vi "prompt_generation.vi"(8 "error in (no error)":errorcluster) -> (0 "error out":errorcluster, 3 "prompt":string)   [LabVIEW 2020]
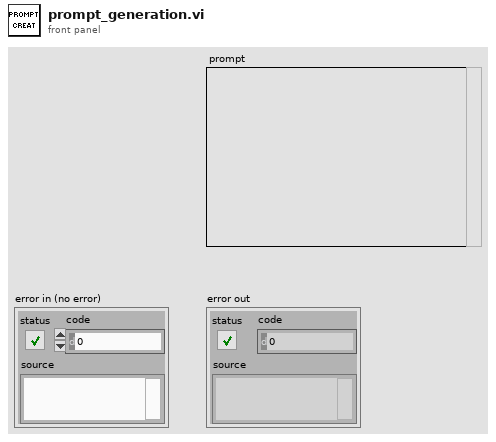
[diagram p1: front panel]
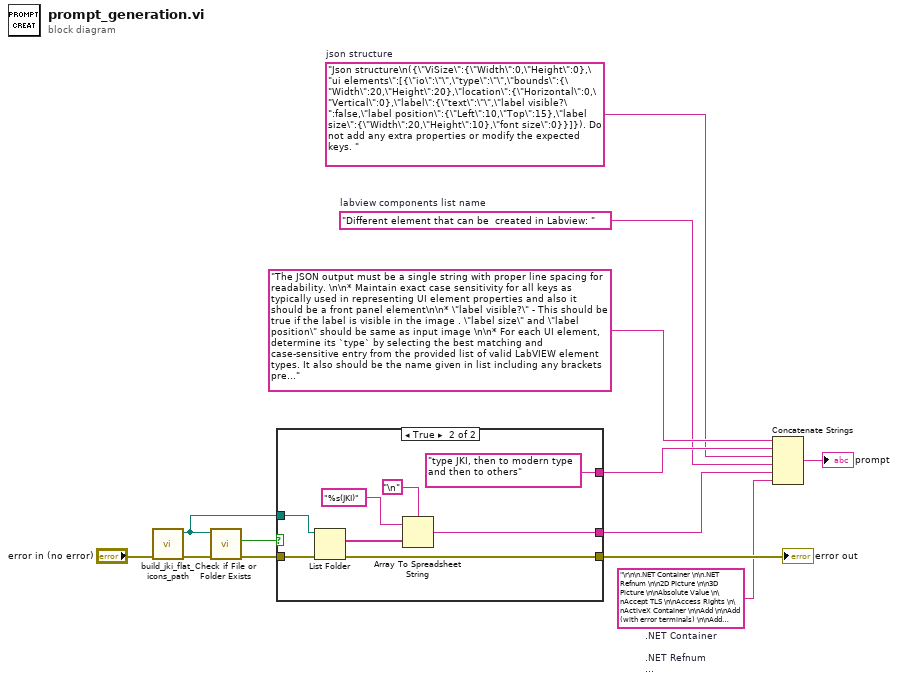
[diagram p0: block diagram]
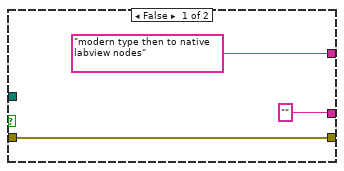
[diagram p2: hidden frame]
diagram:
  w4 = "\r\n\n.NET Container \n\n.NET Refnum \n\n2D Picture \n\n3D Picture \n\nAbsolute Value \n\nAccept TLS \n\nAccess Rights \n\nActiveX Container \n\nAdd \n\nAdd (with error terminals) \n\nAdd Array Elements \n\nAdd Entropy \n\nAdd Private Key To TLS Configuration \n\nAdd Trusted Certificate To TLS Configuration \n\nAgitator \n\nAllSpoll \n\nAlways Copy \n\nAnd \n\nAnd Array Elements \n\nAppend True/False String \n\nApplication Refnum \n\nArray (block diagram constant) \n\nArray (classic) \n\nArray (modern) \n\nArray Interface Control \n\nArray Max & Min \n\nArray of Strings to Path \n\nArray Size \n\nArray Subset \n\nArray To Cluster \n\nArray To Spreadsheet String \n\nArrayMemInfo \n\nAssert Structural Type Match \n\nAssert Structural Type Mismatch \n\nAtmospheric Tank (classic) \n\nAtmospheric Tank (modern) \n\nAutomation Close \n\nAutomation Open \n\nAutomation Refnum \n\nAvogadro Constant (1/mol) \n\nBase 10 Logarithm Of e \n\nBin #1 \n\nBin #2 \n\nBitpack to Array \n\nBluetooth Close Connection \n\nBluetooth Create Listener \n\nBluetooth Discover \n\nBluetooth Network Connection Refnum \n\nBluetooth Open Connection \n\nBluetooth Read \n\nBluetooth Wait On Listener \n\nBluetooth Write \n\nBoolean Array To Number \n\nBoolean To (0,1) \n\nBuild Array \n\nBuild Cluster Array \n\nBuild Map \n\nBuild Matrix \n\nBuild Path \n\nBuild Set \n\nBuild Waveform \n\nBundle \n\nBundle By Name \n\nByte Array To String \n\nByte Array To UTF-8 String \n\nByte Stream File Refnum \n\nCall By Reference \n\nCall Chain \n\nCall Library Function Node \n\nCall Parent Class Method \n\nCAN Channel (block diagram constant) \n\nCAN Channel (classic) \n\nCAN Channel (modern) \n\nCAN Channel (system) \n\nCAN Interface (block diagram constant) \n\nCAN Interface (classic) \n\nCAN Interface (modern) \n\nCAN Interface (system) \n\nCAN Task (block diagram constant) \n\nCAN Task (classic) \n\nCAN Task (modern) \n\nCAN Task (system) \n\nCancel Button (modern) \n\nCancel Button (system) \n\nCancel Notification \n\nCarriage Return Constant \n\nCase Structure \n\nCast Unit Bases \n\nCheck Valve \n\nCheckbox (classic) \n\nCheckBox (modern) \n\nCheckbox (system) \n\nClass Specifier Constant \n\nClassic Color Box \n\nClassic Color Ramp \n\nClassic Horizontal Slide Switch \n\nClassic Vertical Slide \n\nClear Fixed-Point Overflow Status \n\nClose File \n\nClose File (deprecated) \n\nClose Python Session \n\nClose Reference \n\nClose TLS Configuration \n\nClose Variable Connection \n\nClosure Structure \n\nCluster (classic) \n\nCluster (modern) \n\nCluster Constant \n\nCluster To Array \n\nCode Interface Node \n\nCoerce To Type \n\nCollection Size \n\nColor Box Constant \n\nColor Box Thin Border \n\nColored Rectangle (broken?) \n\nCombo Box (classic) \n\nCombo Box (modern) \n\nCombo Box (system) \n\nCombo Box Constant \n\nComplex Conjugate \n\nComplex To Polar \n\nComplex To Re/Im \n\nCompound Arithmetic \n\nCompressor \n\nConcatenate Strings \n\nConditional Disable Structure \n\nConstructor Node \n\nControl & Simulation Loop \n\nControl Help Window \n\nControl Online Help \n\nControl Refnum \n\nConvert Unit \n\nConveyer \n\nCopy \n\nCopy (deprecated) \n\nCosecant \n\nCosine \n\nCotangent \n\nCPU Information \n\nCreate Folder \n\nCreate Network Stream Endpoint \n\nCreate Network Stream Reader Endpoint \n\nCreate Network Stream Writer Endpoint \n\nCreate Stream \n\nCreate Unique Network Stream Endpoint \n\nCreate Unique Network Stream Reader Endpoint \n\nCreate Unique Network Stream Writer Endpoint \n\nCreate User Event \n\nCurrent Processor ID \n\nCurrent VI's Menubar \n\nCurrent VI's Path \n\nDAQmx Analog Trigger Source (block diagram constant) \n\nDAQmx Analog Trigger Source (classic) \n\nDAQmx Analog Trigger Source (modern) \n\nDAQmx Analog Trigger Source (system) \n\nDAQmx Device Name (block diagram constant) \n\nDAQmx Device Name (classic) \n\nDAQmx Device Name (modern) \n\nDAQmx Device Name (system) \n\nDAQmx Global Channel (block diagram constant) \n\nDAQmx Global Channel (classic) \n\nDAQmx Global Channel (modern) \n\nDAQmx Global Channel (system) \n\nDAQmx Physical Channel (block diagram constant) \n\nDAQmx Physical Channel (classic) \n\nDAQmx Physical Channel (modern) \n\nDAQmx Physical Channel (system) \n\nDAQmx Scale Name (block diagram constant) \n\nDAQmx Scale Name (classic) \n\nDAQmx Scale Name (modern) \n\nDAQmx Scale Name (system) \n\nDAQmx Switch (block diagram constant) \n\nDAQmx Switch (classic) \n\nDAQmx Switch (modern) \n\nDAQmx Switch (system) \n\nDAQmx Task Name (block diagram constant) \n\nDAQmx Task Name (classic) \n\nDAQmx Task Name (modern) \n\nDAQmx Task Name (system) \n\nDAQmx Terminal (block diagram constant) \n\nDAQmx Terminal (classic) \n\nDAQmx Terminal (modern) \n\nDAQmx Terminal (system) \n\nData Cache Size \n\nData Log File Refnum \n\nData Value Reference \n\nData Value Reference Constant \n\nDataSocket Close \n\nDataSocket Open \n\nDataSocket Read \n\nDataSocket Refnum \n\nDataSocket Write \n\nDate/Time To Seconds \n\nDecimal Digit? \n\nDecimal String To Number \n\nDecimate 1D Array \n\nDecomposeLockDataValRef \n\nDecomposeVariant \n\nDecrement \n\nDefault Directory \n\nDelete \n\nDelete (deprecated) \n\nDelete Data Value Reference \n\nDelete From Array \n\nDelete Menu Items \n\nDelete Variant Attribute \n\nDelete Waveform Attribute \n\nDeny Access \n\nDequeue Element \n\nDestroy Stream Endpoint \n\nDestroy User Event \n\nDevClear \n\nDevClearList \n\nDevice Control/Status \n\nDevice Refnum \n\nDiagram Disable Structure \n\nDial (classic) \n\nDial (modern) \n\nDigital Data (classic) \n\nDigital Data (modern) \n\nDigital Waveform Graph (classic) \n\nDigital Waveform Graph (modern) \n\nDirect Variable Read \n\nDirect Variable Write \n\nDivide \n\nDivide (with error terminals) \n\nDlg Horiz Scrollbar \n\nDlg Mac Group Box \n\nDlg Numeric #1 \n\nDlg Numeric #2 \n\nDlg String \n\nDlg Vert Scrollbar \n\nDown Arrow \n\nDown Bow Valve (flat) \n\nDown Bow Valve (outline) \n\nDown Bow Valve (shaded) \n\nDown Rect Valve (flat) \n\nDown Rect Valve (outline) \n\nDown Rect Valve (shaded) \n\nDown Tee (flat) \n\nDown Tee (shaded) \n\nDynamic FPGA Interface Cast \n\nEased Corner Rectangle \n\nElement of Set? \n\nElementary Charge (C) \n\nEmpty Array? \n\nEmpty Collection? \n\nEmpty Path Constant \n\nEmpty String Constant \n\nEmpty String/Path? \n\nEnable Menu Tracking \n\nEnableLocal \n\nEnableRemote \n\nEnd of Line Constant \n\nEnqueue Element \n\nEnqueue Element At Opposite End \n\nEnum (classic) \n\nEnum (modern) \n\nEnum (system) \n\nEnum Constant \n\nEOF \n\nEqual To 0? \n\nEqual? \n\nError Ring Constant \n\nEvent Callback Refnum \n\nEvent Data Node \n\nEvent Structure \n\nExchanger \n\nExclusive Or \n\nExponential \n\nExponential (Arg) -1 \n\nExpression Node \n\nFalse Constant \n\nFeedback Node \n\nFieldPoint IO Point (block diagram constant) \n\nFieldPoint IO Point (classic) \n\nFieldPoint IO Point (modern) \n\nFIFO Refnum \n\nFile Dialog \n\nFile Dialog (deprecated) \n\nFile Path Control (classic) \n\nFile Path Control (modern) \n\nFile Path Control (system) \n\nFile Path Indicator (classic) \n\nFile Path Indicator (modern) \n\nFile/Directory Info \n\nFile/Directory Info (deprecated) \n\nFindLstn \n\nFindRQS \n\nFirst Call? \n\nFixed-Point Overflow? \n\nFixed-Point to Integer Cast \n\nFlat Box \n\nFlat Circle \n\nFlat Down Triangle \n\nFlat Frame \n\nFlat Left Triangle \n\nFlat Right Triangle \n\nFlat Round Button \n\nFlat Rounded Box \n\nFlat Sequence Structure \n\nFlat Square Button \n\nFlat Up Triangle \n\nFlatten To JSON \n\nFlatten To String \n\nFlatten To XML \n\nFlattened String To Variant \n\nFloating Point Equal? \n\nFlush Event Queue \n\nFlush File \n\nFlush File (deprecated) \n\nFlush Queue \n\nFlush Stream \n\nFor Loop \n\nFork \n\nFormat Date/Time String \n\nFormat Into File \n\nFormat Into String \n\nFormat Value \n\nFormula Node \n\nFPGA Refnum to Session \n\nFract/Exp String To Number \n\nFramed Color Box (classic) \n\nFramed Color Box (modern) \n\nFree Label \n\nFurnace \n\nGauge (classic) \n\nGauge (modern) \n\nGauge for Simon \n\nGenerate Front Panel Activity \n\nGenerate Occurrence \n\nGenerate User Event \n\nGenerate User-Defined Trace Event \n\nGet Control Values by Index \n\nGet Datalog Position \n\nGet Date/Time In Seconds \n\nGet Date/Time String \n\nGet Drag Drop Data \n\nGet File Position \n\nGet File Size \n\nGet Fixed-Point Components \n\nGet Help Window Status \n\nGet Matrix Diagonal \n\nGet Matrix Elements \n\nGet Menu Item Info \n\nGet Menu Selection \n\nGet Menu Short Cut Info \n\nGet Notifier Status \n\nGet Number of Records \n\nGet Permissions \n\nGet Queue Status \n\nGet Submatrix \n\nGet Type and Creator \n\nGet Variant Attribute \n\nGet Volume Info \n\nGet Waveform Attribute \n\nGet Waveform Components \n\nGlobal Variable \n\nGPIB Clear \n\nGPIB Initialization \n\nGPIB Misc \n\nGPIB Read \n\nGPIB Serial Poll \n\nGPIB Status \n\nGPIB Trigger \n\nGPIB Wait \n\nGPIB Write \n\nGravitational Constant (N m2/kg2) \n\nGreater Or Equal To 0? \n\nGreater Or Equal? \n\nGreater Than 0? \n\nGreater? \n\nHandle Peek \n\nHandle Poke \n\nHex Digit? \n\nHexadecimal String To Number \n\nHopper #1 \n\nHopper #2 \n\nHoriz Line \n\nHoriz Pipe (flat) \n\nHoriz Pipe (shaded) \n\nHorizontal Button Box \n\nHorizontal Fill Slide (classic) \n\nHorizontal Fill Slide (modern) \n\nHorizontal Gradient Oval \n\nHorizontal Gradient Rectangle \n\nHorizontal Gradient Rounded Rectangle \n\nHorizontal Graduated Bar \n\nHorizontal Pointer Slide (classic) \n\nHorizontal Pointer Slide (modern) \n\nHorizontal Pointer Slide (system) \n\nHorizontal Progress Bar (modern) \n\nHorizontal Progress Bar (system) \n\nHorizontal Scrollbar \n\nHorizontal Slide (classic) \n\nHorizontal Slide (system) \n\nHorizontal Smooth Box \n\nHorizontal Splitter Bar \n\nHorizontal Splitter Bar (Classic) \n\nHorizontal Splitter Bar (NXG Style) \n\nHorizontal Splitter Bar (System) \n\nHorizontal Switch \n\nHorizontal Tank \n\nHorizontal Toggle Switch (classic) \n\nHorizontal Toggle Switch (modern) \n\nHyperbolic Cosecant \n\nHyperbolic Cosine \n\nHyperbolic Cotangent \n\nHyperbolic Secant \n\nHyperbolic Sine \n\nHyperbolic Tangent \n\nIMAQ Session \n\nImplies \n\nIn Place Element Structure \n\nIn Range and Coerce \n\nInclude Fixed-Point Overflow Status \n\nIncrement \n\nIndex & Bundle Cluster Array \n\nIndex Array \n\nIndex String Array \n\nInitialize Array \n\nInline C Node \n\nInsert Into Array \n\nInsert Into Map \n\nInsert Into Set \n\nInsert Menu Items \n\nInteger to Fixed-Point Cast \n\nIntensity Chart (classic) \n\nIntensity Chart (modern) \n\nIntensity Graph (classic) \n\nIntensity Graph (modern) \n\nInterleave 1D Arrays \n\nInterpolate 1D Array \n\nInverse Cosecant \n\nInverse Cosine \n\nInverse Cotangent \n\nInverse Hyperbolic Cosecant \n\nInverse Hyperbolic Cosine \n\nInverse Hyperbolic Cotangent \n\nInverse Hyperbolic Secant \n\nInverse Hyperbolic Sine \n\nInverse Hyperbolic Tangent \n\nInverse Secant \n\nInverse Sine \n\nInverse Tangent \n\nInverse Tangent (2 Input) \n\nInvoke Node \n\nIP To String \n\nIrDA Close Connection \n\nIrDA Create Listener \n\nIrDA Discover \n\nIrDA Network Connection Refnum \n\nIrDA Open Connection \n\nIrDA Read \n\nIrDA Wait On Listener \n\nIrDA Write \n\nIsDebuggingActive \n\nIVI Delete Session \n\nIVI Logical Name (block diagram constant) \n\nIVI Logical Name (classic) \n\nIVI Logical Name (modern) \n\nIVI New Session \n\nJoin \n\nJoin Numbers \n\nJunction \n\nKnob (classic) \n\nKnob (modern) \n\nLabel (modern) \n\nLabel (system) \n\nLabeled Oblong Button \n\nLabeled Rectangular Button \n\nLabeled Round Button \n\nLabeled Square Button \n\nLabVIEW Object \n\nLeak Variant Value Reference \n\nLED Button \n\nLeft Arrow \n\nLeft Bow Valve (flat) \n\nLeft Bow Valve (outline) \n\nLeft Bow Valve (shaded) \n\nLeft Down Elbow (flat) \n\nLeft Down Elbow (shaded) \n\nLeft Pump (flat) \n\nLeft Pump (shaded) \n\nLeft Rect Valve (flat) \n\nLeft Rect Valve (outline) \n\nLeft Rect Valve (shaded) \n\nLeft Tee (flat) \n\nLeft Tee (shaded) \n\nLeft Up Elbow (flat) \n\nLeft Up Elbow (shaded) \n\nLess Or Equal To 0? \n\nLess Or Equal? \n\nLess Than 0? \n\nLess? \n\nLexical Class \n\nLine (chiseled, system) \n\nLine (chiseled, thick) \n\nLine (chiseled, thin) \n\nLine (thick) \n\nLine (thin) \n\nLine Feed Constant \n\nLine with Arrow (thick) \n\nLine with Arrow (thin) \n\nList Directory \n\nList Folder \n\nListbox (classic) \n\nListbox (modern) \n\nListbox (system) \n\nListbox Symbol Ring Constant \n\nLoad Certificates Into Memory \n\nLoad Private Key Into Memory \n\nLocal Variable \n\nLock Range \n\nLogarithm Base 10 \n\nLogarithm Base 2 \n\nLogarithm Base X \n\nLogical Shift \n\nLook In Map \n\nLookup Channel Probe \n\nLossy Enqueue Element \n\nLowered Box (thick) \n\nLowered Rounded Box \n\nMachine Epsilon \n\nMake TLS Configuration Immutable \n\nMakeAddr \n\nMantissa & Exponent \n\nMap \n\nMap Constant \n\nMatch First String \n\nMatch Pattern \n\nMatch True/False String \n\nMathScript Call By Reference \n\nMathScript Node \n\nMATLAB script \n\nMatrix Size \n\nMax & Min \n\nMenu Refnum \n\nMenu Ring (classic) \n\nMenu Ring (modern) \n\nMenu-Popup Ring \n\nMerge Errors \n\nMerge Signals \n\nMeter (classic) \n\nMeter (modern) \n\nMixed Checkbox (system) \n\nMixed Signal Graph \n\nMolar Gas Constant (J/(mol K)) \n\nMotion Resource (block diagram constant) \n\nMotion Resource (classic) \n\nMotion Resource (modern) \n\nMotor (flat) \n\nMotor (shaded) \n\nMove \n\nMove (deprecated) \n\nMulti-Segment Pipe \n\nMulticolumn Listbox (classic) \n\nMulticolumn Listbox (modern) \n\nMulticolumn Listbox (system) \n\nMultiply \n\nMultiply (with error terminals) \n\nMultiply Array Elements \n\nMultirate Structure \n\nNatural Logarithm \n\nNatural Logarithm (Arg +1) \n\nNatural Logarithm Base \n\nNatural Logarithm Of 10 \n\nNatural Logarithm Of 2 \n\nNatural Logarithm Of Pi \n\nNegate \n\nNegative Infinity \n\nNew Data Value Reference \n\nNew Directory \n\nNew File \n\nNew TLS Configuration \n\nNew VI \n\nNew VI Object \n\nNot \n\nNot A Number/Path/Refnum? \n\nNot A Path Constant \n\nNot a Refnum Constant \n\nNot a Shared Variable \n\nNot And \n\nNot Equal To 0? \n\nNot Equal? \n\nNot Exclusive Or \n\nNot Or \n\nNotifier Refnum \n\nNumber of Cache Levels \n\nNumber To Boolean Array \n\nNumber To Decimal String \n\nNumber To Engineering String \n\nNumber To Exponential String \n\nNumber To Fractional String \n\nNumber To Hexadecimal String \n\nNumber To Octal String \n\nNumeric Constant \n\nNumeric Control (classic) \n\nNumeric Control (modern) \n\nNumeric Control (system) \n\nNumeric Indicator (classic) \n\nNumeric Indicator (modern) \n\nObtain Notifier \n\nObtain Queue \n\nOccurrence Refnum \n\nOctal Digit? \n\nOctal String To Number \n\nOK Button (modern) \n\nOK Button (system) \n\nOld VISA Open \n\nOLE Variant \n\nOne Button Dialog \n\nOpen and Verify Variable Connection \n\nOpen Application Reference \n\nOpen Device \n\nOpen Dynamic Bitfile Reference \n\nOpen File \n\nOpen Python Session \n\nOpen Tank (flat classic) \n\nOpen Tank (shaded classic) \n\nOpen Variable Connection \n\nOpen Variable Connection in Background \n\nOpen VI Object Reference \n\nOpen VI Reference \n\nOpen/Create/Replace Datalog \n\nOpen/Create/Replace File \n\nOr \n\nOr Array Elements \n\nOval with Shadow \n\nPackage Matrix \n\nPassControl \n\nPath Constant \n\nPath to Array of Strings \n\nPath To String \n\nPath Type \n\nPi \n\nPi Divided By 2 \n\nPi Multiplied By 2 \n\nPick Line \n\nPict Ring (classic) \n\nPict Ring (modern) \n\nPict Ring (system) \n\nPixMap \n\nPixMap (warning: dangerous) \n\nPlanck's Constant (J/Hz) \n\nPlatform Flat Square Button \n\nPlug-In Control \n\nPolar To Complex \n\nPolar To Re/Im \n\nPositive Infinity \n\nPower Of 10 \n\nPower Of 2 \n\nPower Of X \n\nPPoll \n\nPPollConfig \n\nPPollUnconfig \n\nPreallocated Read from Binary File \n\nPreserve Run-Time Class \n\nPressure Tank (flat) \n\nPressure Tank (shaded) \n\nPreview Queue Element \n\nPrintable? \n\nProperty Node \n\nPulldown Menu Ring \n\nPush Button \n\nPython Node \n\nPython Session Refnum \n\nQueue Refnum \n\nQuit LabVIEW \n\nQuotient & Remainder \n\nRace Structure \n\nRadio Button (system) \n\nRadio Buttons (classic) \n\nRadio Buttons (modern) \n\nRadio Buttons (system) \n\nRaised Box (classic) \n\nRaised Box (modern) \n\nRaised Circle \n\nRaised Down Triangle \n\nRaised Frame \n\nRaised Left Triangle \n\nRaised Right Triangle \n\nRaised Rounded Box \n\nRaised Up Triangle \n\nRandom Number (0-1) \n\nRcvRespMsg \n\nRe-accept TLS \n\nRe/Im To Complex \n\nRe/Im To Polar \n\nRead Datalog \n\nRead Device \n\nRead File \n\nRead from Binary File \n\nRead from Text File \n\nRead Map Max & Min Keys \n\nRead Multiple Elements from Stream \n\nRead Set Max & Min \n\nRead Single Element from Stream \n\nRead Variable \n\nRead Variable with Timeout \n\nReadStatus \n\nReceive \n\nReceiveSetup \n\nRecessed Box \n\nRecessed Circle \n\nRecessed Down Triangle \n\nRecessed Frame (modern) \n\nRecessed Frame (system) \n\nRecessed Left Triangle \n\nRecessed Menu Ring \n\nRecessed Right Triangle \n\nRecessed Rounded Box \n\nRecessed Up Triangle \n\nReciprocal \n\nReciprocal Of e \n\nReciprocal Of Pi \n\nRecomposeUnlockDataValRef (warning: dangerous) \n\nRecomposeVariant (warning: dangerous) \n\nRectangular Stop Button \n\nRefnum to Path \n\nRefnum to Session \n\nRegion \n\nRegister Event Callback \n\nRegister For Events \n\nRegister Session \n\nRelease Notifier \n\nRelease Queue \n\nRemove Fixed-Point Overflow Status \n\nRemove From Map \n\nRemove From Set \n\nReplace Array Subset \n\nReplace Substring \n\nRequest Deallocation \n\nResetSys \n\nReshape Array \n\nResize Matrix \n\nResource Index \n\nReverse 1D Array \n\nReverse String \n\nRight Arrow \n\nRight Bow Valve (flat) \n\nRight Bow Valve (outline) \n\nRight Bow Valve (shaded) \n\nRight Down Elbow (flat) \n\nRight Down Elbow (shaded) \n\nRight Pump (flat) \n\nRight Pump (shaded) \n\nRight Rect Valve (flat) \n\nRight Rect Valve (outline) \n\nRight Rect Valve (shaded) \n\nRight Tee (flat) \n\nRight Tee (shaded) \n\nRight Up Elbow (flat) \n\nRight Up Elbow (shaded) \n\nRocker \n\nRotary Feeder \n\nRotate \n\nRotate 1D Array \n\nRotate Left With Carry \n\nRotate Right With Carry \n\nRotate String \n\nRound Button \n\nRound LED (classic) \n\nRound LED (modern) \n\nRound Light \n\nRound Push Button \n\nRound Push Button (profile) \n\nRound Radio Button \n\nRound Stop Button \n\nRound To Nearest \n\nRound Toward +Infinity \n\nRound Toward -Infinity \n\nRounded Rectangle with Shadow \n\nRT FIFO Create \n\nRT FIFO Delete \n\nRT FIFO Read \n\nRT FIFO Write \n\nRydberg Constant (1/m) \n\nScale By Power Of 2 \n\nScan From File \n\nScan From String \n\nScan String For Tokens \n\nScan Value \n\nScanned Variable Read \n\nScanned Variable Write \n\nSearch 1D Array \n\nSearch and Replace String \n\nSearch Variable Container \n\nSearch/Split String \n\nSecant \n\nSeconds To Date/Time \n\nSeek \n\nSelect \n\nSend \n\nSend Notification \n\nSendCmds \n\nSendDataBytes \n\nSendIFC \n\nSendList \n\nSendLLO \n\nSendSetup \n\nSession to Refnum \n\nSet \n\nSet Constant \n\nSet Control Values by Index \n\nSet Datalog Position \n\nSet File Position \n\nSet File Size \n\nSet Matrix Diagonal \n\nSet Matrix Elements \n\nSet Menu Item Info \n\nSet Number of Records \n\nSet Occurrence \n\nSet Permissions \n\nSet Submatrix \n\nSet Type and Creator \n\nSet Variant Attribute \n\nSet Waveform Attribute \n\nSetRWLS \n\nSetTimeOut \n\nShared Variable \n\nShared Variable Constant \n\nShared Variable Control (classic) \n\nShared Variable Control (modern) \n\nShared Variable to String \n\nSign \n\nSimple Horizontal Slide \n\nSimple Numeric \n\nSimple String \n\nSimple Vertical Slide \n\nSinc \n\nSine \n\nSine & Cosine \n\nSize Handle \n\nSlide Switch \n\nSmoothed Oval \n\nSmoothed Rounded Rectangle \n\nSort 1D Array \n\nSort Array of String \n\nSpeed Of Light In Vacuum (m/sec) \n\nSpin Control (system) \n\nSplit 1D Array \n\nSplit Button \n\nSplit Number \n\nSplit Signals \n\nSpreadsheet String To Array \n\nSquare \n\nSquare Button \n\nSquare LED (classic) \n\nSquare LED (modern) \n\nSquare Light \n\nSquare Push Button \n\nSquare Push Button (profile) \n\nSquare Radio Button \n\nSquare Root \n\nStacked Sequence Structure \n\nStart TLS \n\nState \n\nState Diagram \n\nStatic VI Reference \n\nStop \n\nStop Button \n\nString Constant \n\nString Control (classic) \n\nString Control (modern) \n\nString Control (system) \n\nString Indicator (classic) \n\nString Indicator (modern) \n\nString Length \n\nString Subset \n\nString To Byte Array \n\nString To IP \n\nString To Path \n\nString to Shared Variable \n\nStrip Path \n\nSubPanel \n\nSubPanel (Classic) \n\nSubPanel (NXG Style) \n\nSubPanel (System) \n\nSubtract \n\nSubtract (with error terminals) \n\nSwap Bytes \n\nSwap Values \n\nSwap Vector Element \n\nSwap Words \n\nTab Constant \n\nTab Control (classic) \n\nTab Control (modern) \n\nTab Control (NXG Style) \n\nTab Control (system) \n\nTable (classic) \n\nTable (modern) \n\nTable (system) \n\nTag Attribute Ring \n\nTangent \n\nTank (classic) \n\nTank (modern) \n\nTarget Structure \n\nTCP Close Connection \n\nTCP Create Listener \n\nTCP Flattened Read \n\nTCP Flattened Write \n\nTCP Flex Read \n\nTCP Flex Write \n\nTCP Network Connection Refnum \n\nTCP Open Connection \n\nTCP Read \n\nTCP Wait On Listener \n\nTCP Write \n\nTDMS Advanced Asynchronous Read (Data Ref) \n\nTDMS Advanced Asynchronous Write (Data Ref) \n\nTDMS Close \n\nTDMS Configure Asynchronous Reads (Data Ref) \n\nTDMS Configure Asynchronous Writes (Data Ref) \n\nTDMS Defragment \n\nTDMS Delete Data \n\nTDMS File \n\nTDMS Flush \n\nTDMS Get Asynchronous Read Status (Data Ref) \n\nTDMS Get Asynchronous Write Status (Data Ref) \n\nTDMS Get Properties \n\nTDMS In Memory Close \n\nTDMS In Memory Open \n\nTDMS In Memory Read Bytes \n\nTDMS List Contents \n\nTDMS Open \n\nTDMS Read \n\nTDMS Refnum To File ID \n\nTDMS Set Properties \n\nTDMS Write \n\nTDMS Write IP \n\nTemporary Directory \n\nTestSRQ \n\nTestSys \n\nText & Pict Ring (classic) \n\nText & Pict Ring (modern) \n\nText Button \n\nText Ring (block diagram constant) \n\nText Ring (classic) \n\nText Ring (modern) \n\nText Ring (system) \n\nText to UTF-8 \n\nThermometer (classic) \n\nThermometer (modern) \n\nThreshold 1D Array \n\nTick Count (ms) \n\nTime Stamp (block diagram constant) \n\nTime Stamp Control (classic) \n\nTime Stamp Control (modern) \n\nTime Stamp Control (system) \n\nTime Stamp Indicator (classic) \n\nTime Stamp Indicator (modern) \n\nTimed Loop \n\nTimed Sequence \n\nTLS configuration \n\nTLS Connection? \n\nTo Byte Integer \n\nTo Double Precision Complex \n\nTo Double Precision Float \n\nTo Extended Precision Complex \n\nTo Extended Precision Float \n\nTo Fixed-Point \n\nTo Long Integer \n\nTo Lower Case \n\nTo More Generic Class \n\nTo More Specific Class \n\nTo OLE Variant \n\nTo Probe String \n\nTo Quad Integer \n\nTo Single Precision Complex \n\nTo Single Precision Float \n\nTo Time Stamp \n\nTo Unsigned Byte Integer \n\nTo Unsigned Long Integer \n\nTo Unsigned Quad Integer \n\nTo Unsigned Word Integer \n\nTo Upper Case \n\nTo Variant \n\nTo Word Integer \n\nTraditional DAQ Channel (block diagram constant) \n\nTraditional DAQ Channel (classic) \n\nTraditional DAQ Channel (modern) \n\nTranspose 1D Array \n\nTranspose 2D Array \n\nTranspose Matrix \n\nTree (classic) \n\nTree (modern) \n\nTree (system) \n\nTrigger \n\nTriggerList \n\nTwo Button Dialog \n\nType and Creator \n\nType Cast \n\nType Error \n\nType Must Be Array \n\nType Must Be Cluster \n\nType Of \n\nType Specialization Structure \n\nUDP Close \n\nUDP Multicast Open \n\nUDP Network Connection Refnum \n\nUDP Open \n\nUDP Read \n\nUDP Write \n\nUnbitpack from Array \n\nUnbundle \n\nUnbundle By Name \n\nUnflatten From JSON \n\nUnflatten From String \n\nUnflatten From XML \n\nUnleak Variant Value Reference \n\nUnpackage Matrix \n\nUnregister For Events \n\nUnregister Session \n\nUp Arrow \n\nUp Bow Valve (flat) \n\nUp Bow Valve (outline) \n\nUp Bow Valve (shaded) \n\nUp Rect Valve (flat) \n\nUp Rect Valve (outline) \n\nUp Rect Valve (shaded) \n\nUp Tee (flat) \n\nUp Tee (shaded) \n\nUser Defined Refnum \n\nUser Defined Refnum Tag (block diagram constant) \n\nUser Defined Refnum Tag (classic) \n\nUser Defined Refnum Tag (modern) \n\nUser Defined Refnum Tag Flatten (classic) \n\nUser Defined Refnum Tag Flatten (modern) \n\nUser Defined Tag (block diagram constant) \n\nUser Defined Tag (classic) \n\nUser Defined Tag (modern) \n\nUser Item \n\nUTF-8 String To Byte Array \n\nUTF-8 to Text \n\nVariable Class Specifier Constant \n\nVariable Name Constant \n\nVariant \n\nVariant To Data \n\nVariant To Flattened String \n\nVert Line \n\nVert Pipe (flat) \n\nVert Pipe (shaded) \n\nVert Rocker \n\nVertical Fill Slide (classic) \n\nVertical Fill Slide (modern) \n\nVertical Gradient Oval \n\nVertical Gradient Rectangle \n\nVertical Gradient Rounded Rectangle \n\nVertical Graduated Bar \n\nVertical Pointer Slide (classic) \n\nVertical Pointer Slide (modern) \n\nVertical Pointer Slide (system) \n\nVertical Progress Bar (modern) \n\nVertical Progress Bar (system) \n\nVertical Scrollbar \n\nVertical Slide (system) \n\nVertical Slide Switch (classic) \n\nVertical Slide Switch (modern) \n\nVertical Smooth Box \n\nVertical Splitter Bar \n\nVertical Splitter Bar (Classic) \n\nVertical Splitter Bar (NXG Style) \n\nVertical Splitter Bar (System) \n\nVertical Switch \n\nVertical Toggle Switch (classic) \n\nVertical Toggle Switch (modern) \n\nVI Library \n\nVI Refnum \n\nVI Server Reference \n\nVISA Assert Interrupt Signal \n\nVISA Assert Trigger \n\nVISA Assert Utility Signal \n\nVISA Clear \n\nVISA Close \n\nVISA Disable Event \n\nVISA Discard Events \n\nVISA Enable Event \n\nVISA Find Resource \n\nVISA Flush I/O Buffer \n\nVISA GPIB Command \n\nVISA GPIB Control ATN \n\nVISA GPIB Control REN \n\nVISA GPIB Pass Control \n\nVISA GPIB Send IFC \n\nVISA In 16 \n\nVISA In 32 \n\nVISA In 64 \n\nVISA In 8 \n\nVISA Lock \n\nVISA Map Address \n\nVISA Map Trigger \n\nVISA Memory Allocation \n\nVISA Memory Allocation Ex \n\nVISA Memory Free \n\nVISA Move \n\nVISA Move In 16 \n\nVISA Move In 32 \n\nVISA Move In 64 \n\nVISA Move In 8 \n\nVISA Move Out 16 \n\nVISA Move Out 32 \n\nVISA Move Out 64 \n\nVISA Move Out 8 \n\nVISA Open \n\nVISA Out 16 \n\nVISA Out 32 \n\nVISA Out 64 \n\nVISA Out 8 \n\nVISA Peek 16 \n\nVISA Peek 32 \n\nVISA Peek 64 \n\nVISA Peek 8 \n\nVISA Poke 16 \n\nVISA Poke 32 \n\nVISA Poke 64 \n\nVISA Poke 8 \n\nVISA Read \n\nVISA Read STB \n\nVISA Read To File \n\nVISA Refnum to Session \n\nVISA Resource Name \n\nVISA resource name (classic) \n\nVISA resource name (modern) \n\nVISA Set I/O Buffer Size \n\nVISA Status Description \n\nVISA Unlock \n\nVISA Unmap Address \n\nVISA Unmap Trigger \n\nVISA USB Control In \n\nVISA USB Control Out \n\nVISA VXI Cmd or Query \n\nVISA Wait on Event \n\nVISA Write \n\nVISA Write From File \n\nVolume Info \n\nWait (ms) \n\nWait For Activity \n\nWait For Front Panel Activity \n\nWait for GPIB RQS \n\nWait on Notification \n\nWait on Notification from Multiple \n\nWait on Notification from Multiple with Notifier History \n\nWait on Notification with Notifier History \n\nWait on Occurrence \n\nWait Until Next ms Multiple \n\nWaitSRQ \n\nWaveform Chart \n\nWaveform Chart (classic) \n\nWaveform Chart (modern) \n\nWaveform Graph (classic) \n\nWaveform Graph (modern) \n\nWhile Loop #1 \n\nWhile Loop #2 \n\nWhite Space? \n\nWrite Datalog \n\nWrite Device \n\nWrite File \n\nWrite Multiple Elements to Stream \n\nWrite Single Element to Stream \n\nWrite to Binary File \n\nWrite to Text File \n\nWrite Variable \n\nWrite Variable with Timeout \n\nXY Graph (classic) \n\nXY Graph (modern) \n\nY-th Root of X \n\n "  # .NET Container   .NET Refnum   2D Picture   3D Picture   Absolute Value   Accept TLS   Access Rights   ActiveX Container   Add   Add (with error terminals)   Add Array Elements   Add Entropy   Add Private Key To TLS Configuration   Add Trusted Certificate To TLS Configuration   Agitator   AllSpoll   Always Copy   And   And Array Elements   Append True/False String   Application Refnum   Array (block diagram constant)   Array (classic)   Array (modern)   Array Interface Control   Array Max & Min   Array of Strings to Path   Array Size   Array Subset   Array To Cluster   Array To Spreadsheet String   ArrayMemInfo   Assert Structural Type Match   Assert Structural Type Mismatch   Atmospheric Tank (classic)   Atmospheric Tank (modern)   Automation Close   Automation Open   Automation Refnum   Avogadro Constant (1/mol)   Base 10 Logarithm Of e   Bin #1   Bin #2   Bitpack to Array   Bluetooth Close Connection   Bluetooth Create Listener   Bluetooth Discover   Bluetooth Network Connection Refnum   Bluetooth Open Connection   Bluetooth Read   Bluetooth Wait On Listener   Bluetooth Write   Boolean Array To Number   Boolean To (0,1)   Build Array   Build Cluster Array   Build Map   Build Matrix   Build Path   Build Set   Build Waveform   Bundle   Bundle By Name   Byte Array To String   Byte Array To UTF-8 String   Byte Stream File Refnum   Call By Reference   Call Chain   Call Library Function Node   Call Parent Class Method   CAN Channel (block diagram constant)   CAN Channel (classic)   CAN Channel (modern)   CAN Channel (system)   CAN Interface (block diagram constant)   CAN Interface (classic)   CAN Interface (modern)   CAN Interface (system)   CAN Task (block diagram constant)   CAN Task (classic)   CAN Task (modern)   CAN Task (system)   Cancel Button (modern)   Cancel Button (system)   Cancel Notification   Carriage Return Constant   Case Structure   Cast Unit Bases   Check Valve   Checkbox (classic)   CheckBox (modern)   Checkbox (system)   Class Specifier Constant   Classic Color Box   Classic Color Ramp   Classic Horizontal Slide Switch   Classic Vertical Slide   Clear Fixed-Point Overflow Status   Close File   Close File (deprecated)   Close Python Session   Close Reference   Close TLS Configuration   Close Variable Connection   Closure Structure   Cluster (classic)   Cluster (modern)   Cluster Constant   Cluster To Array   Code Interface Node   Coerce To Type   Collection Size   Color Box Constant   Color Box Thin Border   Colored Rectangle (broken?)   Combo Box (classic)   Combo Box (modern)   Combo Box (system)   Combo Box Constant   Complex Conjugate   Complex To Polar   Complex To Re/Im   Compound Arithmetic   Compressor   Concatenate Strings   Conditional Disable Structure   Constructor Node   Control & Simulation Loop   Control Help Window   Control Online Help   Control Refnum   Convert Unit   Conveyer   Copy   Copy (deprecated)   Cosecant   Cosine   Cotangent   CPU Information   Create Folder   Create Network Stream Endpoint   Create Network Stream Reader Endpoint   Create Network Stream Writer Endpoint   Create Stream   Create Unique Network Stream Endpoint   Create Unique Network Stream Reader Endpoint   Create Unique Network Stream Writer Endpoint   Create User Event   Current Processor ID   Current VI's Menubar   Current VI's Path   DAQmx Analog Trigger Source (block diagram constant)   DAQmx Analog Trigger Source (classic)   DAQmx Analog Trigger Source (modern)   DAQmx Analog Trigger Source (system)   DAQmx Device Name (block diagram constant)   DAQmx Device Name (classic)   DAQmx Device Name (modern)   DAQmx Device Name (system)   DAQmx Global Channel (block diagram constant)   DAQmx Global Channel (classic)   DAQmx Global Channel (modern)   DAQmx Global Channel (system)   DAQmx Physical Channel (block diagram constant)   DAQmx Physical Channel (classic)   DAQmx Physical Channel (modern)   DAQmx Physical Channel (system)   DAQmx Scale Name (block diagram constant)   DAQmx Scale Name (classic)   DAQmx Scale Name (modern)   DAQmx Scale Name (system)   DAQmx Switch (block diagram constant)   DAQmx Switch (classic)   DAQmx Switch (modern)   DAQmx Switch (system)   DAQmx Task Name (block diagram constant)   DAQmx Task Name (classic)   DAQmx Task Name (modern)   DAQmx Task Name (system)   DAQmx Terminal (block diagram constant)   DAQmx Terminal (classic)   DAQmx Terminal (modern)   DAQmx Terminal (system)   Data Cache Size   Data Log File Refnum   Data Value Reference   Data Value Reference Constant   DataSocket Close   DataSocket Open   DataSocket Read   DataSocket Refnum   DataSocket Write   Date/Time To Seconds   Decimal Digit?   Decimal String To Number   Decimate 1D Array   DecomposeLockDataValRef   DecomposeVariant   Decrement   Default Directory   Delete   Delete (deprecated)   Delete Data Value Reference   Delete From Array   Delete Menu Items   Delete Variant Attribute   Delete Waveform Attribute   Deny Access   Dequeue Element   Destroy Stream Endpoint   Destroy User Event   DevClear   DevClearList   Device Control/Status   Device Refnum   Diagram Disable Structure   Dial (classic)   Dial (modern)   Digital Data (classic)   Digital Data (modern)   Digital Waveform Graph (classic)   Digital Waveform Graph (modern)   Direct Variable Read   Direct Variable Write   Divide   Divide (with error terminals)   Dlg Horiz Scrollbar   Dlg Mac Group Box   Dlg Numeric #1   Dlg Numeric #2   Dlg String   Dlg Vert Scrollbar   Down Arrow   Down Bow Valve (flat)   Down Bow Valve (outline)   Down Bow Valve (shaded)   Down Rect Valve (flat)   Down Rect Valve (outline)   Down Rect Valve (shaded)   Down Tee (flat)   Down Tee (shaded)   Dynamic FPGA Interface Cast   Eased Corner Rectangle   Element of Set?   Elementary Charge (C)   Empty Array?   Empty Collection?   Empty Path Constant   Empty String Constant   Empty String/Path?   Enable Menu Tracking   EnableLocal   EnableRemote   End of Line Constant   Enqueue Element   Enqueue Element At Opposite End   Enum (classic)   Enum (modern)   Enum (system)   Enum Constant   EOF   Equal To 0?   Equal?   Error Ring Constant   Event Callback Refnum   Event Data Node   Event Structure   Exchanger   Exclusive Or   Exponential   Exponential (Arg) -1   Expression Node   False Constant   Feedback Node   FieldPoint IO Point (block diagram constant)   FieldPoint IO Point (classic)   FieldPoint IO Point (modern)   FIFO Refnum   File Dialog   File Dialog (deprecated)   File Path Control (classic)   File Path Control (modern)   File Path Control (system)   File Path Indicator (classic)   File Path Indicator (modern)   File/Directory Info   File/Directory Info (deprecated)   FindLstn   FindRQS   First Call?   Fixed-Point Overflow?   Fixed-Point to Integer Cast   Flat Box   Flat Circle   Flat Down Triangle   Flat Frame   Flat Left Triangle   Flat Right Triangle   Flat Round Button   Flat Rounded Box   Flat Sequence Structure   Flat Square Button   Flat Up Triangle   Flatten To JSON   Flatten To String   Flatten To XML   Flattened String To Variant   Floating Point Equal?   Flush Event Queue   Flush File   Flush File (deprecated)   Flush Queue   Flush Stream   For Loop   Fork   Format Date/Time String   Format Into File   Format Into String   Format Value   Formula Node   FPGA Refnum to Session   Fract/Exp String To Number   Framed Color Box (classic)   Framed Color Box (modern)   Free Label   Furnace   Gauge (classic)   Gauge (modern)   Gauge for Simon   Generate Front Panel Activity   Generate Occurrence   Generate User Event   Generate User-Defined Trace Event   Get Control Values by Index   Get Datalog Position   Get Date/Time In Seconds   Get Date/Time String   Get Drag Drop Data   Get File Position   Get File Size   Get Fixed-Point Components   Get Help Window Status   Get Matrix Diagonal   Get Matrix Elements   Get Menu Item Info   Get Menu Selection   Get Menu Short Cut Info   Get Notifier Status   Get Number of Records   Get Permissions   Get Queue Status   Get Submatrix   Get Type and Creator   Get Variant Attribute   Get Volume Info   Get Waveform Attribute   Get Waveform Components   Global Variable   GPIB Clear   GPIB Initialization   GPIB Misc   GPIB Read   GPIB Serial Poll   GPIB Status   GPIB Trigger   GPIB Wait   GPIB Write   Gravitational Constant (N m2/kg2)   Greater Or Equal To 0?   Greater Or Equal?   Greater Than 0?   Greater?   Handle Peek   Handle Poke   Hex Digit?   Hexadecimal String To Number   Hopper #1   Hopper #2   Horiz Line   Horiz Pipe (flat)   Horiz Pipe (shaded)   Horizontal Button Box   Horizontal Fill Slide (classic)   Horizontal Fill Slide (modern)   Horizontal Gradient Oval   Horizontal Gradient Rectangle   Horizontal Gradient Rounded Rectangle   Horizontal Graduated Bar   Horizontal Pointer Slide (classic)   Horizontal Pointer Slide (modern)   Horizontal Pointer Slide (system)   Horizontal Progress Bar (modern)   Horizontal Progress Bar (system)   Horizontal Scrollbar   Horizontal Slide (classic)   Horizontal Slide (system)   Horizontal Smooth Box   Horizontal Splitter Bar   Horizontal Splitter Bar (Classic)   Horizontal Splitter Bar (NXG Style)   Horizontal Splitter Bar (System)   Horizontal Switch   Horizontal Tank   Horizontal Toggle Switch (classic)   Horizontal Toggle Switch (modern)   Hyperbolic Cosecant   Hyperbolic Cosine   Hyperbolic Cotangent   Hyperbolic Secant   Hyperbolic Sine   Hyperbolic Tangent   IMAQ Session   Implies   In Place Element Structure   In Range and Coerce   Include Fixed-Point Overflow Status   Increment   Index & Bundle Cluster Array   Index Array   Index String Array   Initialize Array   Inline C Node   Insert Into Array   Insert Into Map   Insert Into Set   Insert Menu Items   Integer to Fixed-Point Cast   Intensity Chart (classic)   Intensity Chart (modern)   Intensity Graph (classic)   Intensity Graph (modern)   Interleave 1D Arrays   Interpolate 1D Array   Inverse Cosecant   Inverse Cosine   Inverse Cotangent   Inverse Hyperbolic Cosecant   Inverse Hyperbolic Cosine   Inverse Hyperbolic Cotangent   Inverse Hyperbolic Secant   Inverse Hyperbolic Sine   Inverse Hyperbolic Tangent   Inverse Secant   Inverse Sine   Inverse Tangent   Inverse Tangent (2 Input)   Invoke Node   IP To String   IrDA Close Connection   IrDA Create Listener   IrDA Discover   IrDA Network Connection Refnum   IrDA Open Connection   IrDA Read   IrDA Wait On Listener   IrDA Write   IsDebuggingActive   IVI Delete Session   IVI Logical Name (block diagram constant)   IVI Logical Name (classic)   IVI Logical Name (modern)   IVI New Session   Join   Join Numbers   Junction   Knob (classic)   Knob (modern)   Label (modern)   Label (system)   Labeled Oblong Button   Labeled Rectangular Button   Labeled Round Button   Labeled Square Button   LabVIEW Object   Leak Variant Value Reference   LED Button   Left Arrow   Left Bow Valve (flat)   Left Bow Valve (outline)   Left Bow Valve (shaded)   Left Down Elbow (flat)   Left Down Elbow (shaded)   Left Pump (flat)   Left Pump (shaded)   Left Rect Valve (flat)   Left Rect Valve (outline)   Left Rect Valve (shaded)   Left Tee (flat)   Left Tee (shaded)   Left Up Elbow (flat)   Left Up Elbow (shaded)   Less Or Equal To 0?   Less Or Equal?   Less Than 0?   Less?   Lexical Class   Line (chiseled, system)   Line (chiseled, thick)   Line (chiseled, thin)   Line (thick)   Line (thin)   Line Feed Constant   Line with Arrow (thick)   Line with Arrow (thin)   List Directory   List Folder   Listbox (classic)   Listbox (modern)   Listbox (system)   Listbox Symbol Ring Constant   Load Certificates Into Memory   Load Private Key Into Memory   Local Variable   Lock Range   Logarithm Base 10   Logarithm Base 2   Logarithm Base X   Logical Shift   Look In Map   Lookup Channel Probe   Lossy Enqueue Element   Lowered Box (thick)   Lowered Rounded Box   Machine Epsilon   Make TLS Configuration Immutable   MakeAddr   Mantissa & Exponent   Map   Map Constant   Match First String   Match Pattern   Match True/False String   MathScript Call By Reference   MathScript Node   MATLAB script   Matrix Size   Max & Min   Menu Refnum   Menu Ring (classic)   Menu Ring (modern)   Menu-Popup Ring   Merge Errors   Merge Signals   Meter (classic)   Meter (modern)   Mixed Checkbox (system)   Mixed Signal Graph   Molar Gas Constant (J/(mol K))   Motion Resource (block diagram constant)   Motion Resource (classic)   Motion Resource (modern)   Motor (flat)   Motor (shaded)   Move   Move (deprecated)   Multi-Segment Pipe   Multicolumn Listbox (classic)   Multicolumn Listbox (modern)   Multicolumn Listbox (system)   Multiply   Multiply (with error terminals)   Multiply Array Elements   Multirate Structure   Natural Logarithm   Natural Logarithm (Arg +1)   Natural Logarithm Base   Natural Logarithm Of 10   Natural Logarithm Of 2   Natural Logarithm Of Pi   Negate   Negative Infinity   New Data Value Reference   New Directory   New File   New TLS Configuration   New VI   New VI Object   Not   Not A Number/Path/Refnum?   Not A Path Constant   Not a Refnum Constant   Not a Shared Variable   Not And   Not Equal To 0?   Not Equal?   Not Exclusive Or   Not Or   Notifier Refnum   Number of Cache Levels   Number To Boolean Array   Number To Decimal String   Number To Engineering String   Number To Exponential String   Number To Fractional String   Number To Hexadecimal String   Number To Octal String   Numeric Constant   Numeric Control (classic)   Numeric Control (modern)   Numeric Control (system)   Numeric Indicator (classic)   Numeric Indicator (modern)   Obtain Notifier   Obtain Queue   Occurrence Refnum   Octal Digit?   Octal String To Number   OK Button (modern)   OK Button (system)   Old VISA Open   OLE Variant   One Button Dialog   Open and Verify Variable Connection   Open Application Reference   Open Device   Open Dynamic Bitfile Reference   Open File   Open Python Session   Open Tank (flat classic)   Open Tank (shaded classic)   Open Variable Connection   Open Variable Connection in Background   Open VI Object Reference   Open VI Reference   Open/Create/Replace Datalog   Open/Create/Replace File   Or   Or Array Elements   Oval with Shadow   Package Matrix   PassControl   Path Constant   Path to Array of Strings   Path To String   Path Type   Pi   Pi Divided By 2   Pi Multiplied By 2   Pick Line   Pict Ring (classic)   Pict Ring (modern)   Pict Ring (system)   PixMap   PixMap (warning: dangerous)   Planck's Constant (J/Hz)   Platform Flat Square Button   Plug-In Control   Polar To Complex   Polar To Re/Im   Positive Infinity   Power Of 10   Power Of 2   Power Of X   PPoll   PPollConfig   PPollUnconfig   Preallocated Read from Binary File   Preserve Run-Time Class   Pressure Tank (flat)   Pressure Tank (shaded)   Preview Queue Element   Printable?   Property Node   Pulldown Menu Ring   Push Button   Python Node   Python Session Refnum   Queue Refnum   Quit LabVIEW   Quotient & Remainder   Race Structure   Radio Button (system)   Radio Buttons (classic)   Radio Buttons (modern)   Radio Buttons (system)   Raised Box (classic)   Raised Box (modern)   Raised Circle   Raised Down Triangle   Raised Frame   Raised Left Triangle   Raised Right Triangle   Raised Rounded Box   Raised Up Triangle   Random Number (0-1)   RcvRespMsg   Re-accept TLS   Re/Im To Complex   Re/Im To Polar   Read Datalog   Read Device   Read File   Read from Binary File   Read from Text File   Read Map Max & Min Keys   Read Multiple Elements from Stream   Read Set Max & Min   Read Single Element from Stream   Read Variable   Read Variable with Timeout   ReadStatus   Receive   ReceiveSetup   Recessed Box   Recessed Circle   Recessed Down Triangle   Recessed Frame (modern)   Recessed Frame (system)   Recessed Left Triangle   Recessed Menu Ring   Recessed Right Triangle   Recessed Rounded Box   Recessed Up Triangle   Reciprocal   Reciprocal Of e   Reciprocal Of Pi   RecomposeUnlockDataValRef (warning: dangerous)   RecomposeVariant (warning: dangerous)   Rectangular Stop Button   Refnum to Path   Refnum to Session   Region   Register Event Callback   Register For Events   Register Session   Release Notifier   Release Queue   Remove Fixed-Point Overflow Status   Remove From Map   Remove From Set   Replace Array Subset   Replace Substring   Request Deallocation   ResetSys   Reshape Array   Resize Matrix   Resource Index   Reverse 1D Array   Reverse String   Right Arrow   Right Bow Valve (flat)   Right Bow Valve (outline)   Right Bow Valve (shaded)   Right Down Elbow (flat)   Right Down Elbow (shaded)   Right Pump (flat)   Right Pump (shaded)   Right Rect Valve (flat)   Right Rect Valve (outline)   Right Rect Valve (shaded)   Right Tee (flat)   Right Tee (shaded)   Right Up Elbow (flat)   Right Up Elbow (shaded)   Rocker   Rotary Feeder   Rotate   Rotate 1D Array   Rotate Left With Carry   Rotate Right With Carry   Rotate String   Round Button   Round LED (classic)   Round LED (modern)   Round Light   Round Push Button   Round Push Button (profile)   Round Radio Button   Round Stop Button   Round To Nearest   Round Toward +Infinity   Round Toward -Infinity   Rounded Rectangle with Shadow   RT FIFO Create   RT FIFO Delete   RT FIFO Read   RT FIFO Write   Rydberg Constant (1/m)   Scale By Power Of 2   Scan From File   Scan From String   Scan String For Tokens   Scan Value   Scanned Variable Read   Scanned Variable Write   Search 1D Array   Search and Replace String   Search Variable Container   Search/Split String   Secant   Seconds To Date/Time   Seek   Select   Send   Send Notification   SendCmds   SendDataBytes   SendIFC   SendList   SendLLO   SendSetup   Session to Refnum   Set   Set Constant   Set Control Values by Index   Set Datalog Position   Set File Position   Set File Size   Set Matrix Diagonal   Set Matrix Elements   Set Menu Item Info   Set Number of Records   Set Occurrence   Set Permissions   Set Submatrix   Set Type and Creator   Set Variant Attribute   Set Waveform Attribute   SetRWLS   SetTimeOut   Shared Variable   Shared Variable Constant   Shared Variable Control (classic)   Shared Variable Control (modern)   Shared Variable to String   Sign   Simple Horizontal Slide   Simple Numeric   Simple String   Simple Vertical Slide   Sinc   Sine   Sine & Cosine   Size Handle   Slide Switch   Smoothed Oval   Smoothed Rounded Rectangle   Sort 1D Array   Sort Array of String   Speed Of Light In Vacuum (m/sec)   Spin Control (system)   Split 1D Array   Split Button   Split Number   Split Signals   Spreadsheet String To Array   Square   Square Button   Square LED (classic)   Square LED (modern)   Square Light   Square Push Button   Square Push Button (profile)   Square Radio Button   Square Root   Stacked Sequence Structure   Start TLS   State   State Diagram   Static VI Reference   Stop   Stop Button   String Constant   String Control (classic)   String Control (modern)   String Control (system)   String Indicator (classic)   String Indicator (modern)   String Length   String Subset   String To Byte Array   String To IP   String To Path   String to Shared Variable   Strip Path   SubPanel   SubPanel (Classic)   SubPanel (NXG Style)   SubPanel (System)   Subtract   Subtract (with error terminals)   Swap Bytes   Swap Values   Swap Vector Element   Swap Words   Tab Constant   Tab Control (classic)   Tab Control (modern)   Tab Control (NXG Style)   Tab Control (system)   Table (classic)   Table (modern)   Table (system)   Tag Attribute Ring   Tangent   Tank (classic)   Tank (modern)   Target Structure   TCP Close Connection   TCP Create Listener   TCP Flattened Read   TCP Flattened Write   TCP Flex Read   TCP Flex Write   TCP Network Connection Refnum   TCP Open Connection   TCP Read   TCP Wait On Listener   TCP Write   TDMS Advanced Asynchronous Read (Data Ref)   TDMS Advanced Asynchronous Write (Data Ref)   TDMS Close   TDMS Configure Asynchronous Reads (Data Ref)   TDMS Configure Asynchronous Writes (Data Ref)   TDMS Defragment   TDMS Delete Data   TDMS File   TDMS Flush   TDMS Get Asynchronous Read Status (Data Ref)   TDMS Get Asynchronous Write Status (Data Ref)   TDMS Get Properties   TDMS In Memory Close   TDMS In Memory Open   TDMS In Memory Read Bytes   TDMS List Contents   TDMS Open   TDMS Read   TDMS Refnum To File ID   TDMS Set Properties   TDMS Write   TDMS Write IP   Temporary Directory   TestSRQ   TestSys   Text & Pict Ring (classic)   Text & Pict Ring (modern)   Text Button   Text Ring (block diagram constant)   Text Ring (classic)   Text Ring (modern)   Text Ring (system)   Text to UTF-8   Thermometer (classic)   Thermometer (modern)   Threshold 1D Array   Tick Count (ms)   Time Stamp (block diagram constant)   Time Stamp Control (classic)   Time Stamp Control (modern)   Time Stamp Control (system)   Time Stamp Indicator (classic)   Time Stamp Indicator (modern)   Timed Loop   Timed Sequence   TLS configuration   TLS Connection?   To Byte Integer   To Double Precision Complex   To Double Precision Float   To Extended Precision Complex   To Extended Precision Float   To Fixed-Point   To Long Integer   To Lower Case   To More Generic Class   To More Specific Class   To OLE Variant   To Probe String   To Quad Integer   To Single Precision Complex   To Single Precision Float   To Time Stamp   To Unsigned Byte Integer   To Unsigned Long Integer   To Unsigned Quad Integer   To Unsigned Word Integer   To Upper Case   To Variant   To Word Integer   Traditional DAQ Channel (block diagram constant)   Traditional DAQ Channel (classic)   Traditional DAQ Channel (modern)   Transpose 1D Array   Transpose 2D Array   Transpose Matrix   Tree (classic)   Tree (modern)   Tree (system)   Trigger   TriggerList   Two Button Dialog   Type and Creator   Type Cast   Type Error   Type Must Be Array   Type Must Be Cluster   Type Of   Type Specialization Structure   UDP Close   UDP Multicast Open   UDP Network Connection Refnum   UDP Open   UDP Read   UDP Write   Unbitpack from Array   Unbundle   Unbundle By Name   Unflatten From JSON   Unflatten From String   Unflatten From XML   Unleak Variant Value Reference   Unpackage Matrix   Unregister For Events   Unregister Session   Up Arrow   Up Bow Valve (flat)   Up Bow Valve (outline)   Up Bow Valve (shaded)   Up Rect Valve (flat)   Up Rect Valve (outline)   Up Rect Valve (shaded)   Up Tee (flat)   Up Tee (shaded)   User Defined Refnum   User Defined Refnum Tag (block diagram constant)   User Defined Refnum Tag (classic)   User Defined Refnum Tag (modern)   User Defined Refnum Tag Flatten (classic)   User Defined Refnum Tag Flatten (modern)   User Defined Tag (block diagram constant)   User Defined Tag (classic)   User Defined Tag (modern)   User Item   UTF-8 String To Byte Array   UTF-8 to Text   Variable Class Specifier Constant   Variable Name Constant   Variant   Variant To Data   Variant To Flattened String   Vert Line   Vert Pipe (flat)   Vert Pipe (shaded)   Vert Rocker   Vertical Fill Slide (classic)   Vertical Fill Slide (modern)   Vertical Gradient Oval   Vertical Gradient Rectangle   Vertical Gradient Rounded Rectangle   Vertical Graduated Bar   Vertical Pointer Slide (classic)   Vertical Pointer Slide (modern)   Vertical Pointer Slide (system)   Vertical Progress Bar (modern)   Vertical Progress Bar (system)   Vertical Scrollbar   Vertical Slide (system)   Vertical Slide Switch (classic)   Vertical Slide Switch (modern)   Vertical Smooth Box   Vertical Splitter Bar   Vertical Splitter Bar (Classic)   Vertical Splitter Bar (NXG Style)   Vertical Splitter Bar (System)   Vertical Switch   Vertical Toggle Switch (classic)   Vertical Toggle Switch (modern)   VI Library   VI Refnum   VI Server Reference   VISA Assert Interrupt Signal   VISA Assert Trigger   VISA Assert Utility Signal   VISA Clear   VISA Close   VISA Disable Event   VISA Discard Events   VISA Enable Event   VISA Find Resource   VISA Flush I/O Buffer   VISA GPIB Command   VISA GPIB Control ATN   VISA GPIB Control REN   VISA GPIB Pass Control   VISA GPIB Send IFC   VISA In 16   VISA In 32   VISA In 64   VISA In 8   VISA Lock   VISA Map Address   VISA Map Trigger   VISA Memory Allocation   VISA Memory Allocation Ex   VISA Memory Free   VISA Move   VISA Move In 16   VISA Move In 32   VISA Move In 64   VISA Move In 8   VISA Move Out 16   VISA Move Out 32   VISA Move Out 64   VISA Move Out 8   VISA Open   VISA Out 16   VISA Out 32   VISA Out 64   VISA Out 8   VISA Peek 16   VISA Peek 32   VISA Peek 64   VISA Peek 8   VISA Poke 16   VISA Poke 32   VISA Poke 64   VISA Poke 8   VISA Read   VISA Read STB   VISA Read To File   VISA Refnum to Session   VISA Resource Name   VISA resource name (classic)   VISA resource name (modern)   VISA Set I/O Buffer Size   VISA Status Description   VISA Unlock   VISA Unmap Address   VISA Unmap Trigger   VISA USB Control In   VISA USB Control Out   VISA VXI Cmd or Query   VISA Wait on Event   VISA Write   VISA Write From File   Volume Info   Wait (ms)   Wait For Activity   Wait For Front Panel Activity   Wait for GPIB RQS   Wait on Notification   Wait on Notification from Multiple   Wait on Notification from Multiple with Notifier History   Wait on Notification with Notifier History   Wait on Occurrence   Wait Until Next ms Multiple   WaitSRQ   Waveform Chart   Waveform Chart (classic)   Waveform Chart (modern)   Waveform Graph (classic)   Waveform Graph (modern)   While Loop #1   While Loop #2   White Space?   Write Datalog   Write Device   Write File   Write Multiple Elements to Stream   Write Single Element to Stream   Write to Binary File   Write to Text File   Write Variable   Write Variable with Timeout   XY Graph (classic)   XY Graph (modern)   Y-th Root of X
  w6 = "Different element that can be  created in Labview: "  # labview components list name
  w7 = "Json structure\n({\"ViSize\":{\"Width\":0,\"Height\":0},\"ui elements\":[{\"io\":\"\",\"type\":\"\",\"bounds\":{\"Width\":20,\"Height\":20},\"location\":{\"Horizontal\":0,\"Vertical\":0},\"label\":{\"text\":\"\",\"label visible?\":false,\"label position\":{\"Left\":10,\"Top\":15},\"label size\":{\"Width\":20,\"Height\":10},\"font size\":0}}]}). Do not add any extra properties or modify the expected keys. "  # json structure
  n1 = call "build_jki_flat_icons_path.vi"("error in (no error)"="error in (no error)") -> ("error out"=w3:errorcluster, "jki flat icon path"=w1:path)  [unwired: 9 in]
  n2 = call <vilib>:"Check if File or Folder Exists.vi"("error in (no error)"=w3, "path"=w1) -> ("error out"=w10:errorcluster, "file or folder exists?"=w11:bool)  [unwired: 7 in, 1 out]
  n3 = case shown="True" w11 {
    tunnel: ["modern type then to native labview nodes" ("f") "type JKI, then to modern type and then to others"] -> w8
    tunnel: w10 -> [w16 w22]
    tunnel: [w16 w23] -> w9
    tunnel: ["" w17] -> w5
    tunnel: w1 -> [_ w21]
    frame False {
    }
    frame True {
      n4 = List Folder(path=w21, error in=w22) -> (filenames=w20:string[], error out=w23:errorcluster)  [unwired: 2 in, 2 out]
      n5 = Array To Spreadsheet String(delimiter (Tab)="\n", array=w20, 3:"%s(JKI)" ("format string")) -> (spreadsheet string=w17:string)
    }
  }
  "error out" <- w9
  n6 = Concatenate Strings("The JSON output must be a single string with proper line spacing for readability. \n\n* Maintain exact case sensitivity for all keys as typically used in representing UI element properties and also it should be a front panel element\n\n* \"label visible?\" - This should be true if the label is visible in the image . \"label size\" and \"label position\" should be same as input image \n\n* For each UI element, determine its `type` by selecting the best matching and case-sensitive entry from the provided list of valid LabVIEW element types. It also should be the name given in list including any brackets present if any\n\n* If a value for a specific key is not applicable to an identified UI element type, set the value to the appropriate default (e.g., `0` for numerical values, `false` for boolean values), but **do not remove the key-value pair**. \n\n* Treat tab controls in the UI as a relevant \"button type\" present in LabVIEW. \n\n* Accurately determine the `bounds` (Width, Height) and `location` (Horizontal, Vertical) of each UI element based on its position and size in the input image. \n\n* The `type` field must correspond to a valid LabVIEW element type. The `io` field must be one of: \"Control\", \"Indicator\" \n\n* Prioritize using the built-in label associated with a LabVIEW control or indicator. Extract the text and size information directly from this label property. Set `\"label visible?\"` to `true` if the built-in label is visible in the image, and position and size accordingly. \n\n* Create a separate \"Label\" element in the JSON only if there is a distinct text label in the UI image that is not directly associated with a control or indicator.  \n\n* Calculate and populate the `\"ViSize\"` (Width, Height) in the JSON root based on the overall dimensions of the UI image. \n\n*For all elements accurately capture their `bounds`, `location`, `\"label position\"`, and `\"label size\"` as they appear in the image.  \n\n* \"label position\" should be similar to the image and user should see it properly\n\n* The priority for choosing type can be given to elements of \n\n", w8, w7, w6, w5, w4) -> (→"prompt":string)
